vi "04.Evd.2_Ask.4.vi"() -> ()   [LabVIEW 2025]
panel:
  out "[(X*Y*Z)/10]":dbl
  out "Absolute value \nof [X+(Y^4)]":dbl
  out "(X^2)+(Y^2)":dbl
  out "Y/X":dbl
  out "1/Y":dbl
  out "1/X":dbl
  out "X+Y":dbl
  in  "Z":dbl
  in  "Y":dbl
  in  "X":dbl
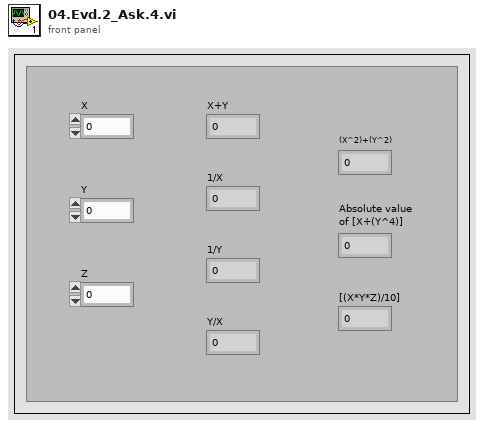
[diagram p1: front panel]
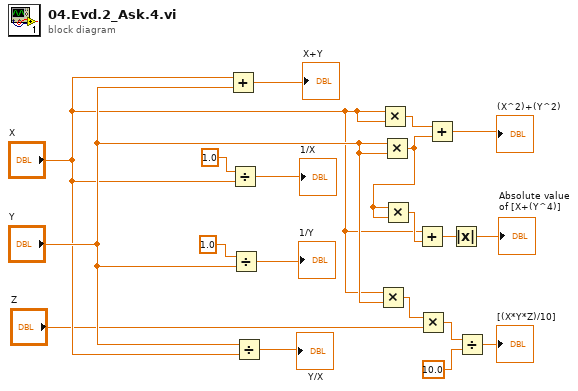
[diagram p0: block diagram]
diagram:
  n1 = Add(x="X", y="Y") -> (x+y=→"X+Y":dbl)
  n2 = Divide(x=1.0, y="X") -> (x/y=→"1/X":dbl)
  n3 = Divide(x=1.0, y="Y") -> (x/y=→"1/Y":dbl)
  n4 = Divide(x="Y", y="X") -> (x/y=→"Y/X":dbl)
  n5 = Multiply(x="X", y="Y") -> (x*y=w5:dbl)
  n6 = Multiply(x="X", y="X") -> (x*y=w13:dbl)
  n7 = Multiply(x="Y", y="Y") -> (x*y=w11:dbl)
  n8 = Multiply(x=w11, y=w11) -> (x*y=w10:dbl)
  n9 = Add(x="X", y=w10) -> (x+y=w9:dbl)
  n10 = Multiply(x=w5, y="Z") -> (x*y=w1:dbl)
  n11 = Add(x=w13, y=w11) -> (x+y=→"(X^2)+(Y^2)":dbl)
  n12 = Absolute Value(x=w9) -> (abs(x)=→"Absolute value \nof [X+(Y^4)]":dbl)
  n13 = Divide(x=w1, y=10.0) -> (x/y=→"[(X*Y*Z)/10]":dbl)
